vi "Final_Project_final_version.vi"() -> ()   [LabVIEW 2015]
uses:
  <vilib>/sound2/lvsound2.llb/Sampling Mode.ctl
  <vilib>/sound2/lvsound2.llb/Sound Output Set Volume (Single).vi
  <vilib>/sound2/lvsound2.llb/Sound Input Read (DBL).vi
  <vilib>/measure/macond.llb/IIR Filter for 1 Chan.vi
  <vilib>/sound2/lvsound2.llb/Sound Output Write (DBL Single).vi
  <vilib>/measure/NI_MAPro.lvlib
panel:
  in  "Sample Rate (Hz)":dbl=22050.0
  in  "Gain":dbl(knob)=9.970820382014532 scale=1.0..10.0
  in  "Master Volume":dbl(knob)=6.346669067478862 scale=0.0..10.0
  in  "Treble":dbl(knob)=0.7901687611998482 scale=0.01..1.0
  in  "Mid":dbl(knob)=0.1981090773084757 scale=0.01..1.0
  in  "Bass":dbl(knob)=0.2048122623560925 scale=0.01..1.0
  in  "Buffer Size (# of samples)":i32=5000
  in  "?":bool
  out "Waveform Graph":waveform(dbl)[](graph)
  # "default = 22050"
  # "Larger buffer gives better quality \nsound, but more playback delay"
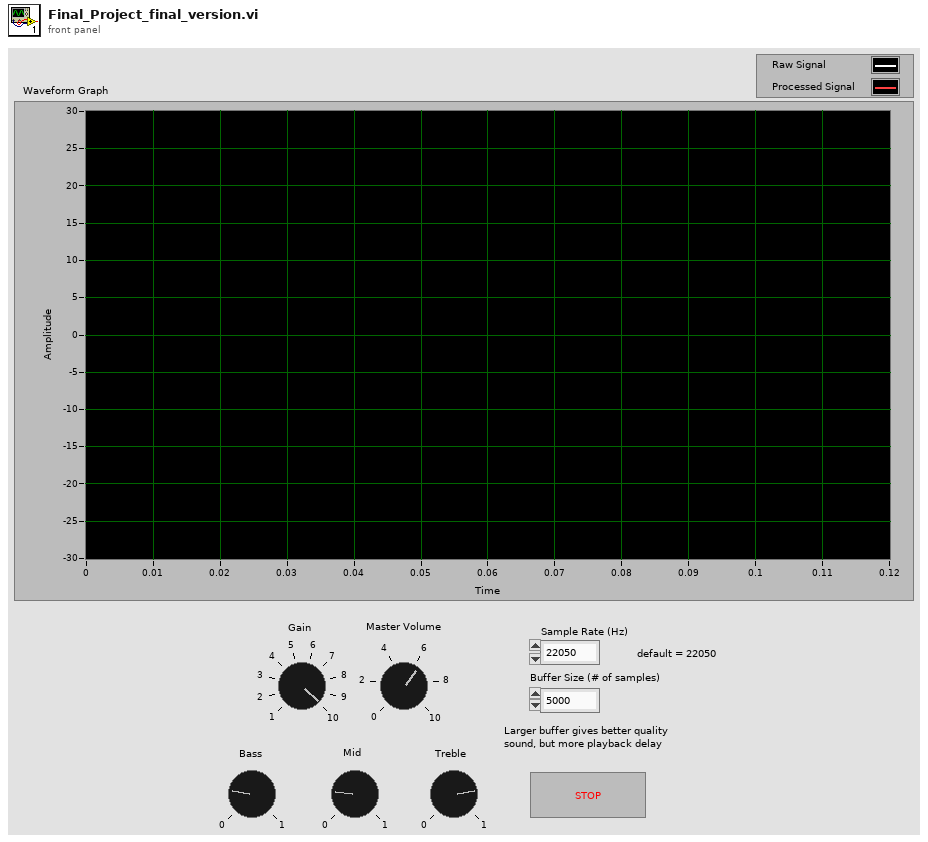
[diagram p1: front panel]
types:
  T1 = typedef "Sampling Mode.ctl" = i32
  T2 = cluster{"Sample Rate (Hz)":dbl, "number of channels":i32, "bits per sample":i32}
  T3 = typedef "Sound Output Task ID.ctl" = u32
  T4 = typedef "Sound Input Task ID.ctl" = u32
  T5 = cluster{"Topology":enum16{"Off", "Butterworth", "Chebyshev", "Inverse Chebyshev", "Elliptic", "Bessel"}, "Type":enum16{"Lowpass", "Highpass", "Bandpass", "Bandstop"}, "Order":i32, "Lower Fc":dbl, "Upper Fc":dbl, "PB Ripple":dbl, "SB Attenuation":dbl}
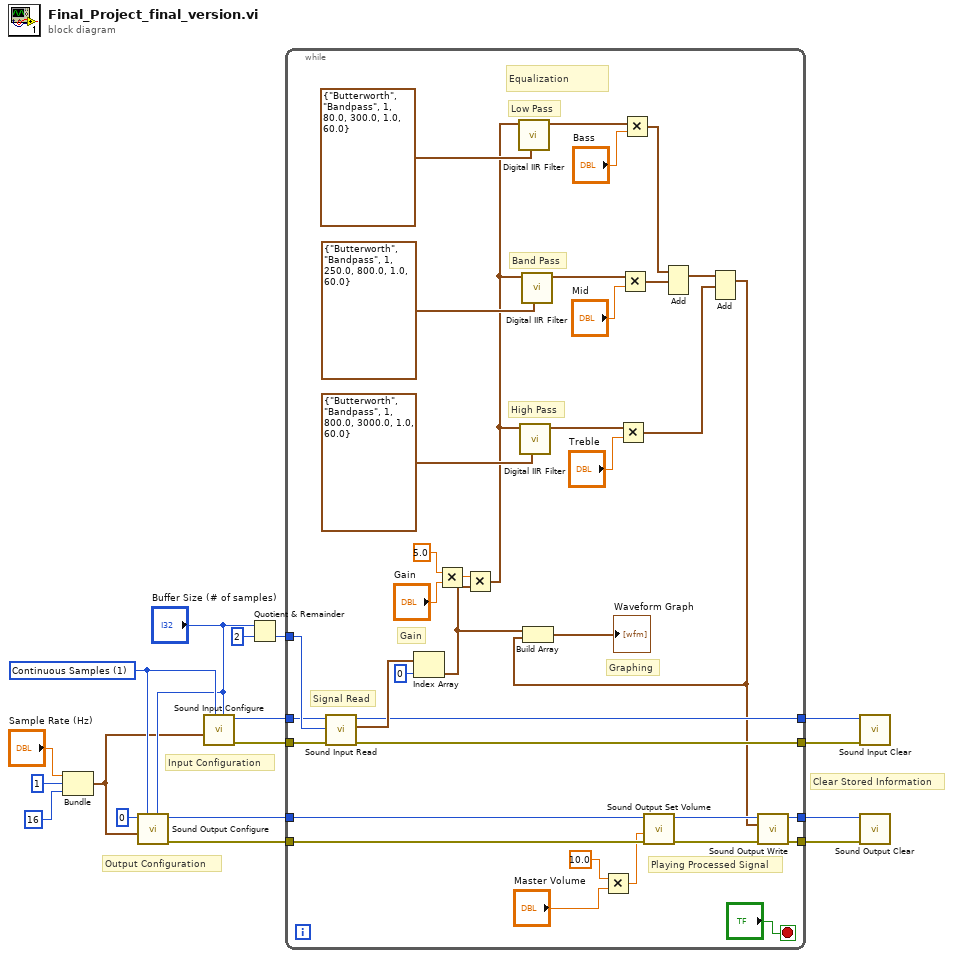
[diagram p0: block diagram]
diagram:
  w17 = T1 1 items=["Finite Samples", "Continuous Samples"] ("sample mode")
  # "Clear Stored Information"
  # "Input Configuration"
  # "Output Configuration"
  n1 = Bundle("Sample Rate (Hz)"="Sample Rate (Hz)", "number of channels"=1, "bits per sample"=16) -> (w2:T2)  [unwired: 1 in]
  n2 = call <vilib>:"Sound Output Configure.vi"("number of samples/ch"="Buffer Size (# of samples)", "sample mode"=w17, "sound format"=w2, "device ID"=u32 0) -> ("error out"=w11:errorcluster, "task ID"=w12:T3)  [unwired: 6 in]
  n3 = call <vilib>:"Sound Input Configure.vi"("number of samples/ch"="Buffer Size (# of samples)", "sample mode"=w17, "sound format"=w2) -> ("error out"=w8:errorcluster, "task ID"=w7:T4)  [unwired: 7 in]
  n4 = Quotient & Remainder(x="Buffer Size (# of samples)", y=2) -> (floor(x/y)=w13:i32)  [unwired: 1 out]
  n5 = while {
    tunnel: w13 -> [w53]
    tunnel: w12 -> [w31]
    tunnel: w11 -> [w29]
    tunnel: [w52] -> w10
    tunnel: [w51] -> w9
    tunnel: w8 -> [w50]
    tunnel: w7 -> [w49]
    tunnel: [w33] -> w5
    tunnel: [w32] -> w6
    stop <- "?" stop-if-true
    # "Playing Processed Signal"
    # "Graphing"
    # "Equalization"
    # "Gain"
    # "Signal Read"
    # "Band Pass"
    # "High Pass"
    # "Low Pass"
    n6 = call-poly <vilib>:"Sound Input Read.vi"("number of samples/ch"=w53, "error in (no error)"=w50, "task ID"=w49) -> ("error out"=w33:errorcluster, "data"=w44:waveform(dbl)[], "task ID out"=w32:T4)  [unwired: 6 in]
    n7 = Index Array(array=w44, index=0) -> (element=w20:waveform(dbl))
    n8 = Multiply(x=5.0, y="Gain") -> (x*y=w22:dbl)
    n9 = Multiply(x=w22, y=w20) -> (x*y=w21:waveform(dbl))
    n10 = call-poly <vilib>:"Digital IIR Filter.vi"("IIR filter specifications"=T5 {"Topology"=enum."Butterworth", "Type"=enum."Bandpass", "Order"=1, "Lower Fc"=80.0, "Upper Fc"=300.0, "PB Ripple"=1.0, "SB Attenuation"=60.0}, "signal in"=w21) -> ("signal out"=w43:waveform(dbl))  [unwired: 7 in, 2 out]
    n11 = call-poly <vilib>:"Digital IIR Filter.vi"("IIR filter specifications"=T5 {"Topology"=enum."Butterworth", "Type"=enum."Bandpass", "Order"=1, "Lower Fc"=800.0, "Upper Fc"=3000.0, "PB Ripple"=1.0, "SB Attenuation"=60.0}, "signal in"=w21) -> ("signal out"=w41:waveform(dbl))  [unwired: 7 in, 2 out]
    n12 = call-poly <vilib>:"Digital IIR Filter.vi"("IIR filter specifications"=T5 {"Topology"=enum."Butterworth", "Type"=enum."Bandpass", "Order"=1, "Lower Fc"=250.0, "Upper Fc"=800.0, "PB Ripple"=1.0, "SB Attenuation"=60.0}, "signal in"=w21) -> ("signal out"=w42:waveform(dbl))  [unwired: 7 in, 2 out]
    n13 = Multiply(x=10.0 ("y"), y="Master Volume") -> (x*y=w25:dbl)
    n14 = Multiply(x=w41, y="Treble") -> (x*y=w37:waveform(dbl))
    n15 = Multiply(x=w42, y="Mid") -> (x*y=w38:waveform(dbl))
    n16 = Multiply(x=w43, y="Bass") -> (x*y=w39:waveform(dbl))
    n17 = call-poly <vilib>:"Sound Output Set Volume.vi"("error in (no error)"=w29, "volume"=w25, "task ID"=w31) -> ("error out"=w28:errorcluster, "task ID out"=w30:T3)  [unwired: 7 in]
    n18 = Add(1:w38, 2:w39) -> (0:w40:waveform(dbl))  [unwired: 1 in, 1 out]
    n19 = Add(1:w37, 2:w40) -> (0:w19:waveform(dbl))  [unwired: 1 in, 1 out]
    n20 = Build Array(w20, w19) -> (→"Waveform Graph":waveform(dbl)[])
    n21 = call-poly <vilib>:"Sound Output Write.vi"("error in (no error)"=w28, "data"=w19, "task ID"=w30) -> ("error out"=w51:errorcluster, "task ID out"=w52:T3)  [unwired: 7 in]
  }
  n22 = call <vilib>:"Sound Input Clear.vi"("error in (no error)"=w5, "task ID"=w6) -> ()  [unwired: 9 in, 1 out]
  n23 = call <vilib>:"Sound Output Clear.vi"("error in (no error)"=w9, "task ID"=w10) -> ()  [unwired: 9 in, 1 out]
